vi "Particle Analysis Report with overlay.vi"() -> ()   [LabVIEW 2016]
doc: "This example introduces the processing area of particle analysis. This example uses the threshold function that converts a grayscale image into a binary image."
uses:
  <vilib>/vision/Image Controls.llb/Overlay Property.ctl
  <vilib>/vision/NI_Vision_Development_Module.lvlib
panel:
  out "Img2":T1(plugin-control)
  out "Img":T1(plugin-control)
  # "Overview: Demonstrates how to use the IMAQ Particle Analysis Report function with a binary image to return information about each particle.\nRequirements: Vision Development Software.\nInstructions:\n1. Run the VI.\n2. Change the Selected Particle to update the Selected Particle Report, and overlay the bounding box for the selected particle."
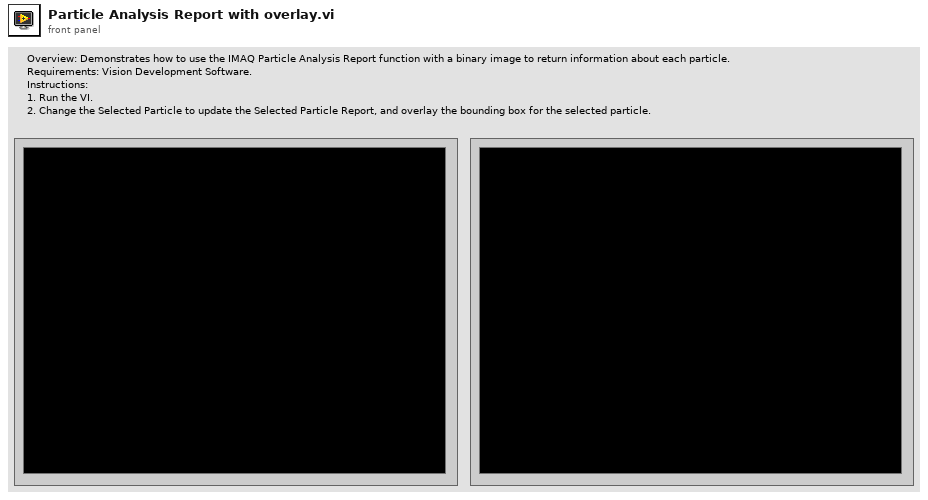
[diagram p1: front panel]
types:
  T1 = typedef "IMAQ Image.ctl" = refnum<image>
  T2 = typedef "Overlay Property.ctl" = cluster{"Property":enum32{"Scale", "Shift", "Rotate", "Symmetry"}, "Behavior":enum32{"Clear", "Keep", "Transform"}}
  T3 = cluster{"Area":dbl, "Number of Holes":dbl, "Bounding Rect":cluster{"Left":dbl, "Top":dbl, "Right":dbl, "Bottom":dbl}, "Center of Mass":cluster{"X":dbl, "Y":dbl}, "Orientation":dbl, "Dimensions":cluster{"Width":dbl, "Height":dbl}}[]
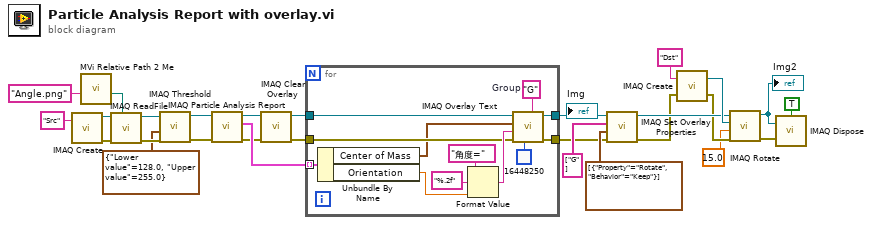
[diagram p0: block diagram]
diagram:
  n1 = call "IMAQ Create"("Image Name"="Src") -> ("New Image"=w27:T1, "error out"=w26:errorcluster)  [unwired: 4 in]
  n2 = call "MVi Relative Path 2 Me.vi"("Relative Path"="Angle.png") -> ("Appended Dir"=w2:path)  [unwired: 5 in, 1 out]
  n3 = call "IMAQ ReadFile"("File Path"=w2, "error in (no error)"=w26, "Image"=w27) -> ("error out"=w24:errorcluster, "Image Out"=w25:T1)  [unwired: 4 in, 3 out]
  n4 = call "IMAQ Threshold"("error in (no error)"=w24, "Range"=cluster{"Lower value":sgl, "Upper value":sgl} {"Lower value"=128.0, "Upper value"=255.0}, "Image Src"=w25) -> ("error out"=w23:errorcluster, "Image Dst Out"=w22:T1)  [unwired: 7 in]
  n5 = call "IMAQ Particle Analysis Report"("error in (no error)"=w23, "Image"=w22) -> ("error out"=w18:errorcluster, "Particle Reports (Pixels)"=w21:T3, "Image Out (duplicate)"=w19:T1)  [unwired: 4 in, 3 out]
  n6 = call "IMAQ Clear Overlay"("error in (no error)"=w18, "Image"=w19) -> ("error out"=w17:errorcluster, "Image Out"=w16:T1)  [unwired: 8 in]
  n7 = for {
    tunnel: w16 -> [w34]
    tunnel: w17 -> [w33]
    tunnel: [w39] -> w13
    tunnel: [w40] -> w6
    tunnel: w21 -> [w35] mode=indexing
    w29 = "G"  # Group
    n8 = Unbundle By Name(w35) -> ("Center of Mass"=w31:cluster{"X":dbl, "Y":dbl}, "Orientation"=w30:dbl)
    n9 = Format Value(string ("")="角度=", format string="%.2f", value (0)=w30) -> (output string=w37:string)
    n10 = call "IMAQ Overlay Text"("Group"=w29, "Text Color (black)"=u32 16448250 ("Color"), "error in (no error)"=w33, "String"=w37, "Origin"=w31, "Image"=w34) -> ("error out"=w39:errorcluster, "Image Out"=w40:T1)  [unwired: 4 in]
  }
  "Img" <- w6
  n11 = call "IMAQ Set Overlay Properties"("Image"=w6, "Groups"=string[] ["G"], "Properties"=T2[] [{"Property"=enum."Rotate", "Behavior"=enum."Keep"}], "error in (no error)"=w13) -> ("Image Out"=w7:T1, "error out"=w5:errorcluster)  [unwired: 4 in]
  n12 = call "IMAQ Create"("Image Name"="Dst", "error in (no error)"=w5) -> ("New Image"=w10:T1, "error out"=w4:errorcluster)  [unwired: 3 in]
  n13 = call "IMAQ Rotate"("error in (no error)"=w4, "Angle (degrees)"=sgl 15.0, "Image Dst"=w10, "Image Src"=w7) -> ("error out"=w12:errorcluster, "Image Dst Out"=w8:T1)  [unwired: 6 in]
  "Img2" <- w8
  n14 = call "IMAQ Dispose"("All Images? (No)"=TRUE, "Image"=w8, "error in (no error)"=w12) -> ()  [unwired: 3 in, 1 out]
